vi "init.vi"(8 "error in (no error)":errorcluster, 11 "ILCTC in":refnum<class "ILCTC.lvclass">) -> (0 "error out":errorcluster, 3 "ILCTC out":refnum<class "ILCTC.lvclass">)   [LabVIEW 2016, in "ILCTC.lvclass"]
uses:
  ILCTC.lvclass
  D:/Code/ts_dcabt/Common_ILC/ILC/ILC.lvclass
  Common_ILC/Configuration/Serial.ctl
  Common_SerialProtocols/Configuration/SerialConfig.ctl
  Common_SerialProtocols/Configuration/SerialProtocol.ctl
  Common_SerialProtocols/Configuration/ProtocolParameters.ctl
  Common_SerialProtocols/Configuration/SerialMessageParameters.ctl
  Common_ILC/Configuration/ADC.ctl
  Common_ILC/Typedefs/ADC Settings.ctl
  Common_ILC/Configuration/Input Channels.ctl
  Common_ILC/Configuration/Scan Rates.ctl
  Common_ILC/ILC/ILC.lvclass/ILC.ctl
  Common_ILC/ILC/ILC.lvclass
  Common_SerialProtocols/SerialProtocols.lvlib
  Common_ILC/Configuration/ILCConfiguration.lvlib
  ConfigurationThisComponent/ConfigurationThisComponent.lvclass
  Common_ILC/Typedefs/ILCTypedefs.lvlib
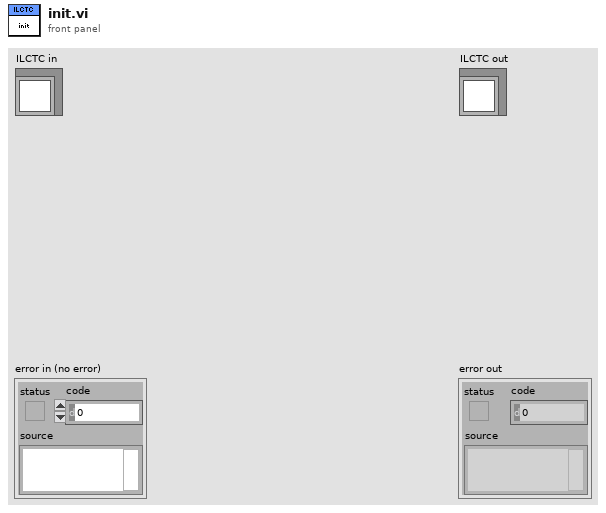
[diagram p1: front panel]
types:
  T1 = typedef "ILCCommon.lvlib/ILCTypedefs.lvlib/ADC Settings.ctl" = cluster{"Input Channels":T2, "Scan Rate (Hz) ":T3, "PGA Gain Coefficient":u8}
  T2 = typedef "ILCCommon.lvlib/ILCConfiguration.lvlib/Input Channels.ctl" = enum16{"Channel 0", "3 Channels", "5 Channels"}
  T3 = typedef "ILCCommon.lvlib/ILCConfiguration.lvlib/Scan Rates.ctl" = enum16{"50", "60", "100", "120", "200", "240", "300", "400", "480", "600", "1200", "2400", "4800"}
  T4 = typedef "ILCCommon.lvlib/ILCConfiguration.lvlib/ADC.ctl" = cluster{"Reference Voltage Vref":dbl[unit], "Nominal Input Range in Counts":u32, "Preamplifier Gain":u8, "Conversion Settling Cycles":u16}
  T5 = typedef "ILCCommon.lvlib/ILCConfiguration.lvlib/Serial.ctl" = cluster{"Serial":T6}
  T6 = typedef "SerialProtocols.lvlib/SerialConfig.ctl" = cluster{"Serial Protocol":T7, "Protocol Parameters":T8, "Serial Message Parameters":T9}
  T7 = typedef "SerialProtocols.lvlib/SerialProtocol.ctl" = enum16{"RS232", "RS485", "SerialSimulator"}
  T8 = typedef "SerialProtocols.lvlib/ProtocolParameters.ctl" = cluster{"VISA resource name":refnum<visa-resource-name>, "Baud Rate":u32, "Data Bits":u16, "Parity":enum16{"None", "Odd", "Even", "Mark", "Space"}, "Flow Control":u16, "Stop Bits":u16, "Timeout (ms)":u32}
  T9 = typedef "SerialProtocols.lvlib/SerialMessageParameters.ctl" = cluster{"Byte Count":u32, "Enable Termination Character":bool, "Termination Char":u8}
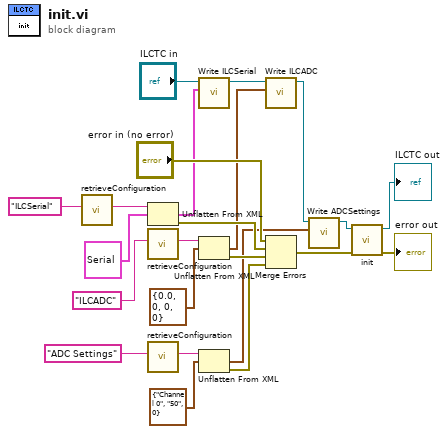
[diagram p0: block diagram]
diagram:
  n1 = call "retrieveConfiguration.vi"("configName"="ILCSerial") -> ("xmlConfig"=w18:string)  [unwired: 8 in, 2 out]
  n2 = Unflatten From XML(xml string=w18, type=T5 {"Serial"={"Serial Protocol"=enum."RS232", "Protocol Parameters"={"VISA resource name"="", "Baud Rate"=0, "Data Bits"=0, "Parity"=enum."None", "Flow Control"=0, "Stop Bits"=0, "Timeout (ms)"=0}, "Serial Message Parameters"={"Byte Count"=0, "Enable Termination Character"=FALSE, "Termination Char"=0}}} ("ILC")) -> (value=w11:T5, error out=w21:errorcluster)  [unwired: 1 in]
  n3 = call "retrieveConfiguration.vi"("configName"="ILCADC") -> ("xmlConfig"=w17:string)  [unwired: 8 in, 2 out]
  n4 = call "retrieveConfiguration.vi"("configName"="ADC Settings") -> ("xmlConfig"=w8:string)  [unwired: 8 in, 2 out]
  n5 = call "Write ILCSerial.vi"("ILC Serial"=w11, "ILC in"="ILCTC in") -> ("ILC out"=w12:refnum<class "ILCTC.lvclass">)  [unwired: 9 in]
  n6 = Unflatten From XML(xml string=w17, type=T4 {"Reference Voltage Vref"=0.0, "Nominal Input Range in Counts"=0, "Preamplifier Gain"=0, "Conversion Settling Cycles"=0} ("ILC ADC")) -> (value=w10:T4, error out=w15:errorcluster)  [unwired: 1 in]
  n7 = Unflatten From XML(xml string=w8, type=T1 {"Input Channels"=enum."Channel 0", "Scan Rate (Hz) "=enum."50", "PGA Gain Coefficient"=0} ("ADC Settings")) -> (value=w1:T1, error out=w6:errorcluster)  [unwired: 1 in]
  n8 = call "Write ILCADC.vi"("ILC ADC"=w10, "ILC in"=w12) -> ("ILC out"=w5:refnum<class "ILCTC.lvclass">)  [unwired: 9 in]
  n9 = Merge Errors("error in (no error)", w21, w15, w6) -> (w9:errorcluster)
  n10 = call "Write ADCSettings.vi"("ADC Settings"=w1, "ILC in"=w5) -> ("ILC out"=w4:refnum<class "ILCTC.lvclass">)  [unwired: 9 in]
  n11 = call-parent "init.vi"("error in (no error)"=w9, "ILC in"=w4) -> ("error out"=→"error out":errorcluster, "ILC out"=→"ILCTC out":refnum<class "ILCTC.lvclass">)  [unwired: 8 in]
